vi "IO_18V7TankControl.vi"(8 "error in":errorcluster, 9 "Speed":i16, 10 "Fill!Drain":bool, 11 "VISA Refnum in":refnum<visa-resource-name>) -> (0 "error out":errorcluster, 1 "Level PV":dbl(slide)=7.1220598220825195 scale=0.0..10.0, 2 "Laser Raw":sgl=2.4953, 3 "VISA Refnum out":refnum<visa-resource-name>)   [LabVIEW 2024]
uses:
  Keyance Demo Code/Keyence LK-G3000/Keyence LK-G3000.lvlib
panel:
  out "TX Buf":string="D0\r"
  out "read buffer ASC":string="!1\r\n"
  # "Use this Timer section\nto measure the Level dl/dt"
  # "Laser ON When Laser\nis on Line."
  # "Use if off line to generate\na test Reply to Write msg"
  # "Target Speed for PWC OLS = 0.52\"/min\nWhich is Speed set to ~17% which 24Vdc"
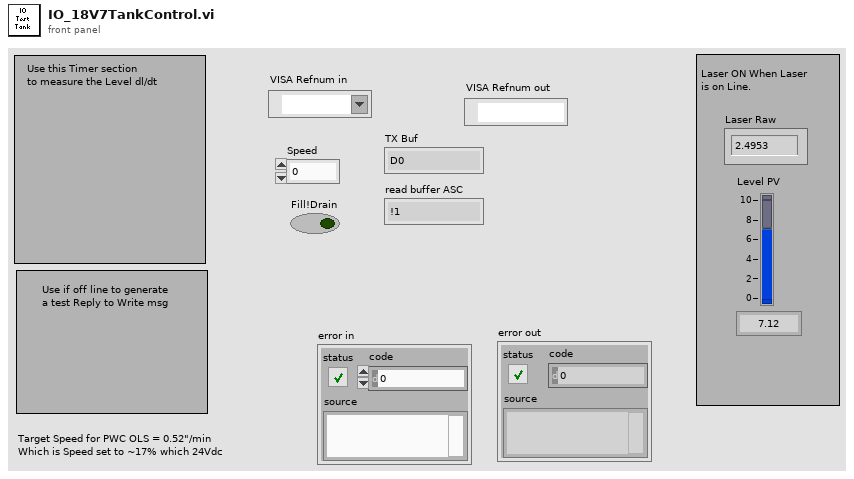
[diagram p1: front panel]
types:
  T1 = cluster{"Fill!Drain":bool, "Speed":i16, "Send Msg":bool, "Write Buf":string}
  T2 = typedef "Keyence LK-G3000.lvlib/LKIF_FLOATVALUE.ctl" = cluster{"LKIF_FLOATRESULT":T3, "Value":sgl}
  T3 = typedef "Keyence LK-G3000.lvlib/LKIF_FLOATRESULT.ctl" = i32
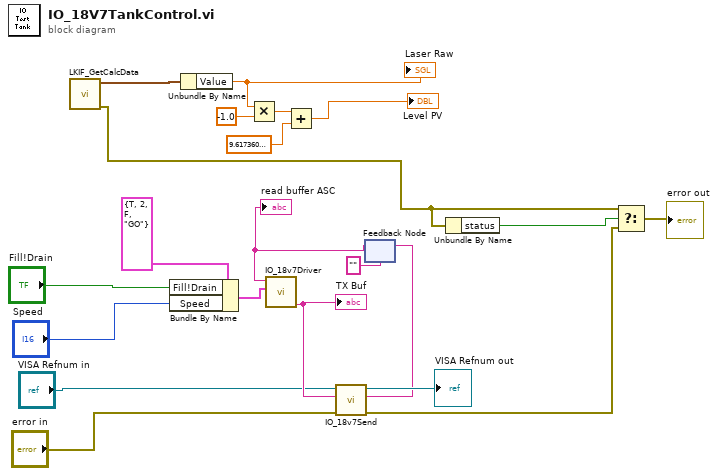
[diagram p0: block diagram]
diagram:
  n1 = call "LKIF_GetCalcData.vi"() -> ("error out"=w2:errorcluster, "CalcData1"=w10:T2)  [unwired: 9 in, 1 out]
  n2 = Bundle By Name(cluster=T1 {"Fill!Drain"=TRUE, "Speed"=2, "Send Msg"=FALSE, "Write Buf"="GO"} ("Inputs"), "Fill!Drain"="Fill!Drain", "Speed"="Speed") -> (w18:T1)
  n3 = Unbundle By Name(w10) -> ("Value"=w9:sgl)
  "Laser Raw" <- w9
  n4 = Multiply(x=w9, y=sgl -1.0) -> (x*y=w7:sgl)
  n5 = Add(x=w7, y=sgl 9.61736) -> (x+y=→"Level PV":sgl)
  n6 = feedback #1("" ("read buffer")) -> (w12:string)
  "read buffer ASC" <- w12
  n7 = call "IO_18v7Driver.vi"("Inputs"=w18, "Reply In"=w12) -> ("Tx Buf Out"=w20:string)  [unwired: 8 in, 1 out]
  "TX Buf" <- w20
  n8 = call "IO_18v7Send.vi"("error in (no error)"="error in", "Tx Buf Out"=w20, "VISA Refnum in"="VISA Refnum in") -> ("error out"=w4:errorcluster, "read buffer"=w13:string, "VISA Refnum out"=→"VISA Refnum out":refnum<visa-resource-name>)  [unwired: 6 in]
  n9 = feedback-in #1(w13) -> ()
  n10 = Unbundle By Name(w2) -> ("status"=w1:bool)
  n11 = Select(t=w2, s=w1, f=w4) -> (s? t:f=→"error out":errorcluster)
